vi "Delete Uint16Array DVR.vi"(8 "error in (no error)":errorcluster, 11 "Uint16Array DVR in":refnum<data-value>) -> (0 "error out":errorcluster, 3 "Uint16Array out":refnum<class "Uint16Array.lvclass">)   [LabVIEW 2013, in "MDSplus.lvlib" / "Uint16Array.lvclass"]
uses:
  <vilib>/MDSplus/Classes/Data_Class/Array_Class/Uint16Array_Class/Uint16Array.lvclass
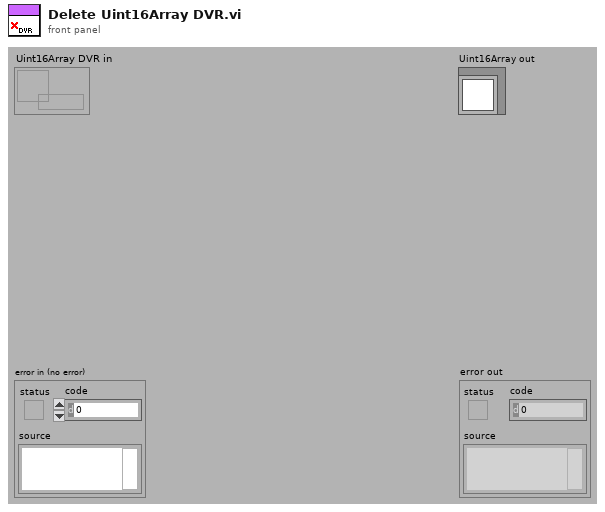
[diagram p1: front panel]
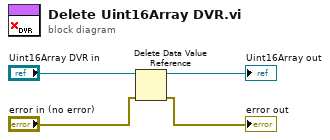
[diagram p0: block diagram]
diagram:
  n1 = Delete Data Value Reference(data value reference="Uint16Array DVR in", error in="error in (no error)") -> (data value=→"Uint16Array out":refnum<class "Uint16Array.lvclass">, error out=→"error out":errorcluster)
